vi "Deform_Mirror_VMap_DUAL_AE.vi"(0 "Mirror ID":string, 1 "Enum":enum16{"WRITE", "READ"}(ring), 7 "V Map In":dbl[][](array[numeric])) -> (8 "V Map Out":dbl[][](array[numeric]))   [LabVIEW 2014]
panel:
  in  "Mirror ID":cluster{"Bottom":dbl[][], "Top":dbl[][]}
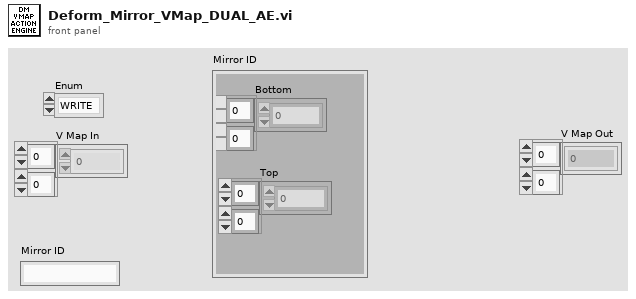
[diagram p1: front panel]
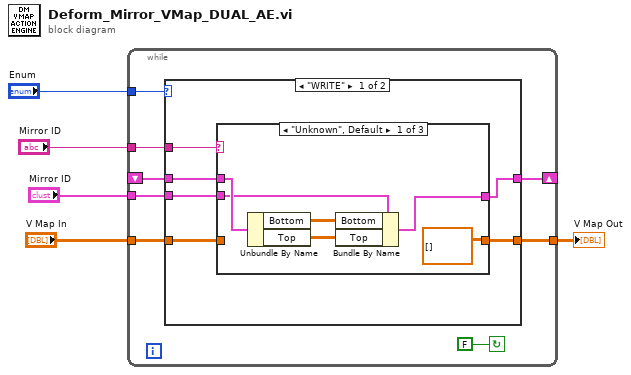
[diagram p0: block diagram]
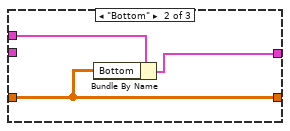
[diagram p2: hidden frame]
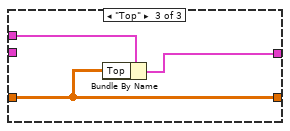
[diagram p3: hidden frame]
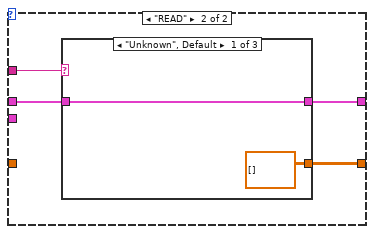
[diagram p4: hidden frame]
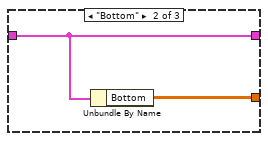
[diagram p5: hidden frame]
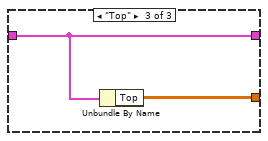
[diagram p6: hidden frame]
diagram:
  n1 = while {
    tunnel: "Enum" -> [w12]
    tunnel: "V Map In" -> [w11]
    tunnel: "Mirror ID" -> [w10]
    shift-right: [w8] -> _
    shift-left: _ -> [w6]
    tunnel: "Mirror ID" -> [w9]
    tunnel: [w7] -> w1
    stop <- FALSE continue-if-true
    n2 = case shown="\"WRITE\"" w12 {
      tunnel: w11 -> [w17 _]
      tunnel: w10 -> [w19 w35]
      tunnel: w9 -> [w18 _]
      tunnel: [w16 w34] -> w8
      tunnel: [w15 w32] -> w7
      tunnel: w6 -> [w14 w33]
      frame "WRITE" {
        n3 = case shown="\"Unknown\", Default" w19 {
          tunnel: w18 -> [w24 _ _]
          tunnel: w17 -> [_ w27 w30]
          tunnel: [w23 w28 w31] -> w16
          tunnel: [dbl[][] [] ("V Map In") w27 w30] -> w15
          tunnel: w14 -> [w25 w26 w29]
          frame "Unknown", Default {
            n4 = Unbundle By Name(w25) -> ("Bottom"=w22:dbl[][], "Top"=w21:dbl[][])
            n5 = Bundle By Name(cluster=w24, "Bottom"=w22, "Top"=w21) -> (w23:cluster{"Bottom":dbl[][], "Top":dbl[][]})
          }
          frame "Bottom" {
            n6 = Bundle By Name(cluster=w26, "Bottom"=w27) -> (w28:cluster{"Bottom":dbl[][], "Top":dbl[][]})
          }
          frame "Top" {
            n7 = Bundle By Name(cluster=w29, "Top"=w30) -> (w31:cluster{"Bottom":dbl[][], "Top":dbl[][]})
          }
        }
      }
      frame "READ" {
        n8 = case shown="\"Unknown\", Default" w35 {
          tunnel: [w37 w39 w41] -> w34
          tunnel: w33 -> [w37 w39 w41]
          tunnel: [dbl[][] [] ("Top") w38 w40] -> w32
          frame "Unknown", Default {
          }
          frame "Bottom" {
            n9 = Unbundle By Name(w39) -> ("Bottom"=w38:dbl[][])
          }
          frame "Top" {
            n10 = Unbundle By Name(w41) -> ("Top"=w40:dbl[][])
          }
        }
      }
    }
  }
  "V Map Out" <- w1
